vi "linFitArrayPress.vi"(1 "volt":sgl[](array[numeric])) -> (0 "press":sgl[](array[numeric]))   [LabVIEW 2021]
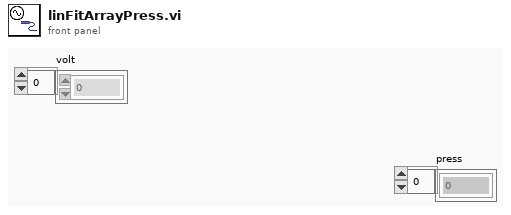
[diagram p1: front panel]
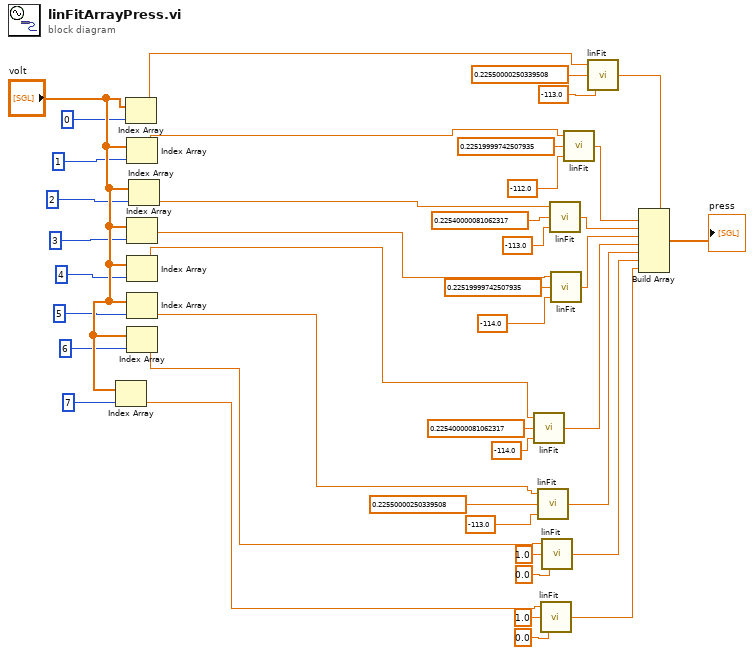
[diagram p0: block diagram]
diagram:
  n1 = Index Array(array="volt", index=7) -> (element=w8:sgl)
  n2 = Index Array(array="volt", index=0) -> (element=w31:sgl)
  n3 = Index Array(array="volt", index=1) -> (element=w24:sgl)
  n4 = Index Array(array="volt", index=3) -> (element=w13:sgl)
  n5 = Index Array(array="volt", index=4) -> (element=w12:sgl)
  n6 = Index Array(array="volt", index=5) -> (element=w10:sgl)
  n7 = Index Array(array="volt", index=6) -> (element=w9:sgl)
  n8 = Index Array(array="volt", index=2) -> (element=w14:sgl)
  n9 = call "linFit.vi"("b"=sgl -114.0, "m"=sgl 0.2254, "x"=w12) -> ("xm+b"=w18:sgl)
  n10 = call "linFit.vi"("b"=sgl -113.0, "m"=sgl 0.2255, "x"=w10) -> ("xm+b"=w17:sgl)
  n11 = call "linFit.vi"("b"=sgl 0.0, "m"=sgl 1.0, "x"=w8) -> ("xm+b"=w2:sgl)
  n12 = call "linFit.vi"("b"=sgl 0.0, "m"=sgl 1.0, "x"=w9) -> ("xm+b"=w16:sgl)
  n13 = call "linFit.vi"("b"=sgl -113.0, "m"=sgl 0.2254, "x"=w14) -> ("xm+b"=w20:sgl)
  n14 = call "linFit.vi"("b"=sgl -114.0, "m"=sgl 0.2252, "x"=w13) -> ("xm+b"=w19:sgl)
  n15 = call "linFit.vi"("b"=sgl -112.0, "m"=sgl 0.2252, "x"=w24) -> ("xm+b"=w21:sgl)
  n16 = call "linFit.vi"("b"=sgl -113.0, "m"=sgl 0.2255, "x"=w31) -> ("xm+b"=w22:sgl)
  n17 = Build Array(w22, w21, w20, w19, w18, w17, w16, w2) -> (→"press":sgl[])
